vi "Graph V50.vi"(0 "valueRef":refnum<vi>, 1 "completeRef":refnum<vi>, 2 "pointsRef":refnum<vi>, 3 "partialRef":refnum<vi>, 4 "error IN":errorcluster) -> (5 "shotGraph":cluster{i32[], sgl[]}[](array[cluster]) {"?" format="%.2f"})   [LabVIEW 2012]
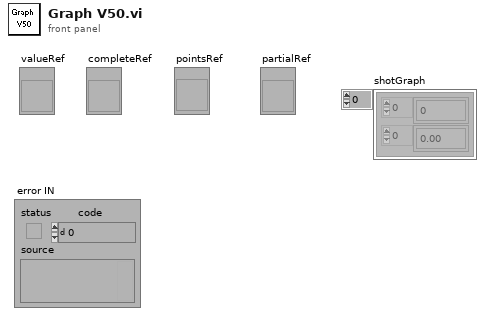
[diagram p1: front panel]
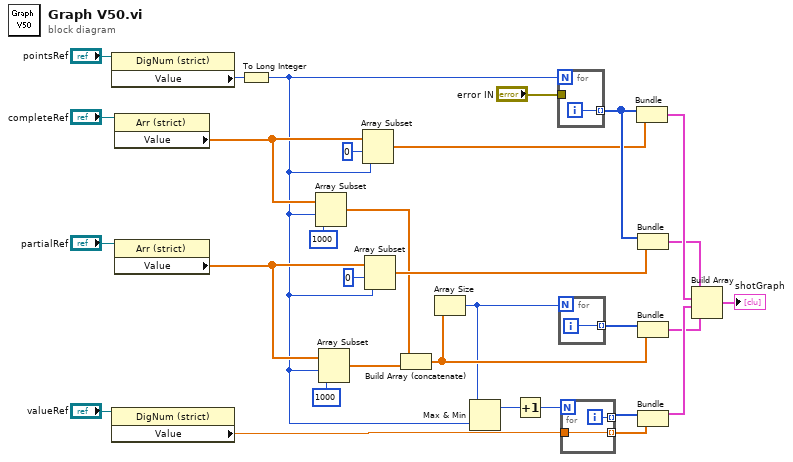
[diagram p0: block diagram]
diagram:
  n1 = property class="DigNum (strict)"(reference="pointsRef") -> ("Value"=w22:i16)  [unwired: 1 in, 2 out]
  n2 = property class="DigNum (strict)"(reference="valueRef") -> ("Value"=w11:sgl)  [unwired: 1 in, 2 out]
  n3 = property class="Arr (strict)"(reference="completeRef") -> ("Value"=w7:sgl[])  [unwired: 1 in, 2 out]
  n4 = property class="Arr (strict)"(reference="partialRef") -> ("Value"=w16:sgl[])  [unwired: 1 in, 2 out]
  n5 = To Long Integer(number=w22) -> (32bit integer=w4:i32)
  n6 = Array Subset(array=w7, index=w4, length=1000 ("Array Length")) -> (w21:sgl[])
  n7 = Array Subset(array=w16, index=w4, length=1000 ("Array Length")) -> (w23:sgl[])
  n8 = Array Subset(array=w7, index=0 ("Array Index"), length=w4) -> (w14:sgl[])
  n9 = Array Subset(array=w16, index=0 ("Array Index"), length=w4) -> (w24:sgl[])
  n10 = Build Array (concatenate)(w21, w23) -> (w28:sgl[])
  n11 = Array Size(array=w28) -> (size(s)=w25:i32)
  n12 = Max & Min(x=w25, y=w4) -> (max(x,y)=w26:i32)  [unwired: 1 out]
  n13 = Increment(x=w26) -> (x+1=w20:i32)
  n14 = for {
    N: w4 -> [_]
    tunnel: [w32] -> w17 mode=indexing
    tunnel: "error IN" -> [_]
    i -> [w32]
  }
  n15 = for {
    N: w25 -> [_]
    tunnel: [w33] -> w15 mode=indexing
    i -> [w33]
  }
  n16 = for {
    N: w20 -> [_]
    tunnel: [w35] -> w13 mode=indexing
    tunnel: w11 -> [w34]
    tunnel: [w34] -> w12 mode=indexing
    i -> [w35]
  }
  n17 = Bundle(w17, w14) -> (w19:cluster{i32[], sgl[]})  [unwired: 1 in]
  n18 = Bundle(w17, w24) -> (w18:cluster{i32[], sgl[]})  [unwired: 1 in]
  n19 = Bundle(w15, w28) -> (w27:cluster{i32[], sgl[]})  [unwired: 1 in]
  n20 = Bundle(w13, w12) -> (w31:cluster{i32[], sgl[]})  [unwired: 1 in]
  n21 = Build Array(w18, w19, w31, w27) -> (→"shotGraph":cluster{i32[], sgl[]}[])
